vi "recycleImage.vi"(8 "error in (no error)":errorcluster, 10 "Video queue":refnum<queue>, 11 "Image pointer recylcing queue":refnum<queue>) -> (0 "error out":errorcluster)   [LabVIEW 2017]
uses:
  <vilib>/vision/Image Controls.llb/IMAQ Image.ctl
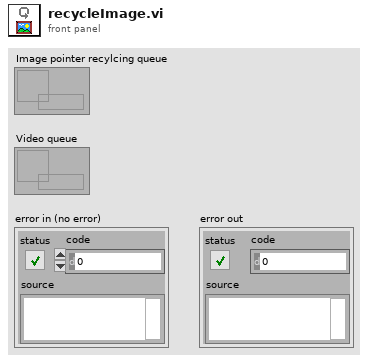
[diagram p1: front panel]
types:
  T1 = typedef "IMAQ Image.ctl" = refnum<image>
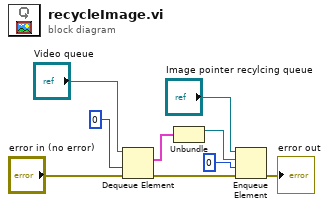
[diagram p0: block diagram]
diagram:
  n1 = Dequeue Element(queue="Video queue", timeout in ms (-1)=0, error in (no error)="error in (no error)") -> (element=w8:cluster{"Image Out":T1, timestamp}, error out=w4:errorcluster)  [unwired: 2 out]
  n2 = Unbundle(w8) -> ("Image Out"=w9:T1)  [unwired: 1 out]
  n3 = Enqueue Element(queue="Image pointer recylcing queue", element=w9, timeout in ms (-1)=0, error in (no error)=w4) -> (error out=→"error out":errorcluster)  [unwired: 2 out]
